vi "Door Closed Interlock Value Change.vi"(8 "error in (no error)":errorcluster, 10 "Door Closed Interlock":bool, 11 "Door Controller in":refnum<class "Door Controller.lvclass">) -> (0 "error out":errorcluster, 3 "Door Controller out":refnum<class "Door Controller.lvclass">)   [LabVIEW 2020, in "Door Controller.lvlib" / "Door Controller.lvclass"]
uses:
  Door Controller.lvclass
  Door Controller.lvclass/Door Controller.ctl
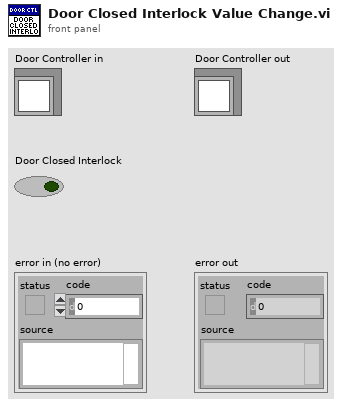
[diagram p1: front panel]
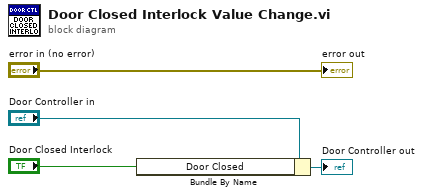
[diagram p0: block diagram]
diagram:
  n1 = Bundle By Name(cluster="Door Controller in", "Door Closed"="Door Closed Interlock") -> (→"Door Controller out":refnum<class "Door Controller.lvclass">)
  "error out" <- "error in (no error)"
